vi "Five Blinking Lights.vi"() -> ()   [LabVIEW 2017]
panel:
  in  "stop":bool
  out "Boolean 5":bool
  out "Boolean 4":bool
  out "Boolean 3":bool
  out "Boolean 2":bool
  out "Boolean":bool
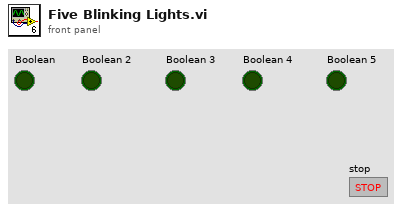
[diagram p1: front panel]
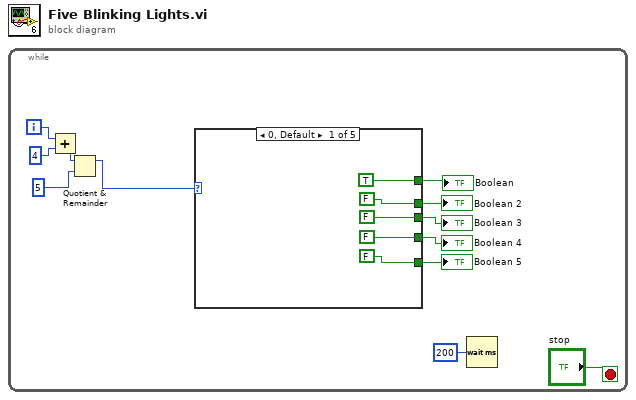
[diagram p0: block diagram]
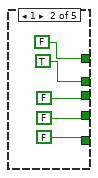
[diagram p2: hidden frame]
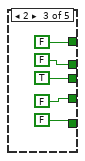
[diagram p3: hidden frame]
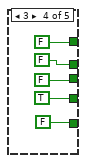
[diagram p4: hidden frame]
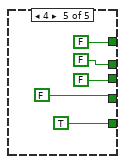
[diagram p5: hidden frame]
diagram:
  n1 = while {
    i -> [w7]
    stop <- "stop" stop-if-true
    n2 = Add(x=w7, y=4) -> (x+y=w6:i32)
    n3 = Quotient & Remainder(x=w6, y=5) -> (x-y*floor(x/y)=w9:i32)  [unwired: 1 out]
    n4 = case shown="0, Default" w9 {
      tunnel: [TRUE FALSE FALSE FALSE FALSE] -> w5
      tunnel: [FALSE TRUE FALSE FALSE FALSE] -> w4
      tunnel: [FALSE FALSE TRUE FALSE FALSE] -> w3
      tunnel: [FALSE FALSE FALSE TRUE FALSE] -> w2
      tunnel: [FALSE FALSE FALSE FALSE TRUE] -> w1
      frame 0, Default {
      }
      frame 1 {
      }
      frame 2 {
      }
      frame 3 {
      }
      frame 4 {
      }
    }
    "Boolean" <- w5
    "Boolean 2" <- w4
    "Boolean 3" <- w3
    "Boolean 4" <- w2
    "Boolean 5" <- w1
    n5 = Wait (ms)(milliseconds to wait=u32 200) -> ()  [unwired: 1 out]
  }
